vi "Check sensor active flag (A).vi"(8 "Error In":errorcluster, 10 "Sensor index":u8, 11 "VISA resource name in":refnum<visa-resource-name>) -> (0 "Error out":errorcluster, 1 "ACK":bool, 2 "Active flag":u8, 3 "VISA resource name out":refnum<visa-resource-name>)   [LabVIEW 2015]
uses:
  Ctls/Cmd str.ctl
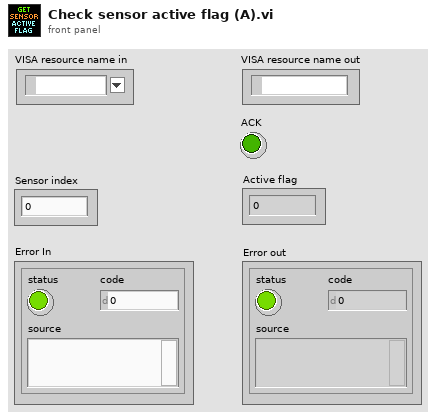
[diagram p1: front panel]
types:
  T1 = typedef "Cmd str.ctl" = string
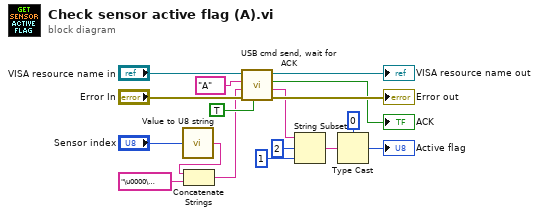
[diagram p0: block diagram]
diagram:
  n1 = call "Value to U8 string.vi"("Value"="Sensor index") -> ("U8 str"=w1:string)
  n2 = Concatenate Strings(w1, "\u0000\u0000\u0000" ("string")) -> (w2:string)
  n3 = call "USB cmd send, wait for ACK.vi"("Wait for ACK?"=TRUE, "Error In"="Error In", "4 byte config str"=w2, "Cmd"=T1 "A", "VISA resource name in"="VISA resource name in") -> ("Error out"=→"Error out":errorcluster, "Return msg"=w9:string, "ACK ok"=→"ACK":bool, "VISA resource name out"=→"VISA resource name out":refnum<visa-resource-name>)  [unwired: 1 in]
  n4 = String Subset(string=w9, offset (0)=2, length (rest)=1 ("length (rest)")) -> (substring=w6:string)
  n5 = Type Cast(type=u8 0 ("length (rest)"), x=w6) -> (*(type *) &x=→"Active flag":u8)
